vi "Measurement Logic.vi"() -> ()   [LabVIEW 2023, in "NIDCPowerSourceDCVoltage.lvlib"]
uses:
  NIDCPowerSourceDCVoltage.lvlib
  Measurement Configuration.ctl
  Measurement Results.ctl
  <vilib>/Plug-In SDKs/Measurements/Measure Call Context/Measure Call Context.lvclass
  <vilib>/gRPC/Generated APIs/ni/measurementlink/discovery/v1/RPC Messages/ni_measurementlink_discovery_v1_ResolveServiceRequest.ctl
  <vilib>/Plug-In SDKs/Clients/Session Management V1/Session Reservation/Session Reservation.lvclass
  <vilib>/Plug-In SDKs/Sessions/niDCPower/NI Session Management niDCPower.lvlib
  NIDCPowerSourceDCVoltage_client/NIDCPowerSourceDCVoltage_client.lvlib
  <vilib>/Plug-In SDKs/Clients/Discovery V1/NI Discovery V1 Client.lvlib
  <vilib>/gRPC/Generated APIs/ni/measurementlink/discovery/v1/ni.measurementlink.discovery.v1.api.lvlib
panel:
  in  "error in":errorcluster
  in  "request data":T1
  out "error out":errorcluster
  out "measure call context out":refnum<class "Measure Call Context.lvclass">
  in  "measure call context in":refnum<class "Measure Call Context.lvclass">
  out "measurement results":T2
  in  "measurement configuration":T3={"pin_names"=[], "voltage_level"=6.0, "voltage_level_range"=6.0, "current_limit"=0.01, "current_limit_range"=0.01, "source_delay"=0.0}
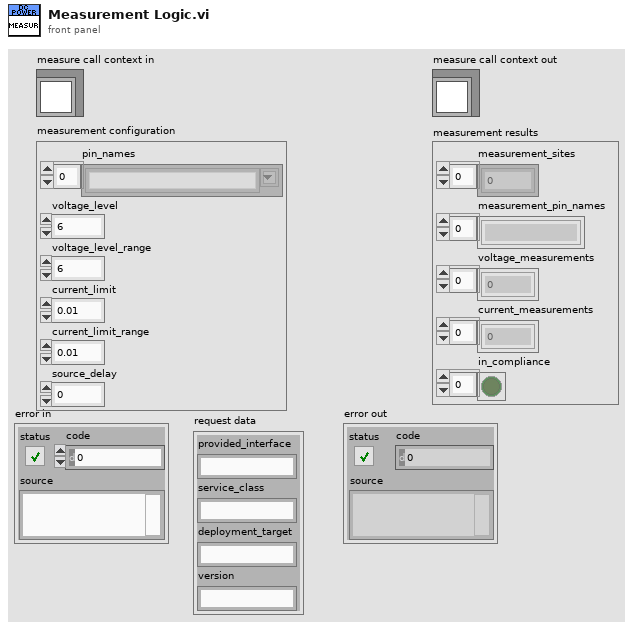
[diagram p1: front panel]
types:
  T1 = typedef "ni.measurementlink.discovery.v1.api.lvlib/ni_measurementlink_discovery_v1_ResolveServiceRequest.ctl" = cluster{"provided_interface":string, "service_class":string, "deployment_target":string, "version":string}
  T2 = typedef "NIDCPowerSourceDCVoltage.lvlib/Measurement Results.ctl" = cluster{"measurement_sites":i32[], "measurement_pin_names":string[], "voltage_measurements":dbl[], "current_measurements":dbl[], "in_compliance":bool[]}
  T3 = typedef "NIDCPowerSourceDCVoltage.lvlib/Measurement Configuration.ctl" = cluster{"pin_names":string[], "voltage_level":dbl, "voltage_level_range":dbl, "current_limit":dbl, "current_limit_range":dbl, "source_delay":dbl}
  T4 = typedef "ni.measurementlink.discovery.v1.api.lvlib/ni_measurementlink_discovery_v1_ServiceLocation.ctl" = cluster{"location":string, "insecure_port":string, "ssl_authenticated_port":string}
  T5 = typedef "grpc-lvsupport-release.lvlib/grpcId.ctl" = u64
  T6 = typedef "NI Session Management niDCPower.lvlib/Connection with Session.ctl" = cluster{"connection":T7, "session":refnum<k15>}
  T7 = typedef "NI Session Management V1 Client.lvlib/Session Reservation.lvclass/Connection.ctl" = cluster{"pin or relay name":string, "site":i32, "instrument type id":string, "channel":string}
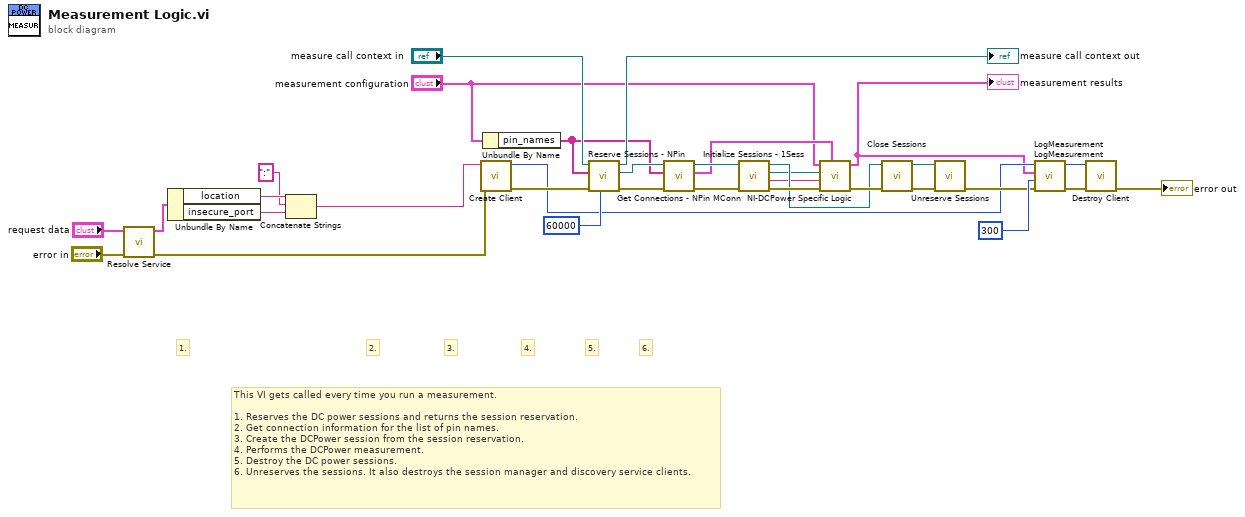
[diagram p0: block diagram]
diagram:
  # "6."
  # "This VI gets called every time you run a measurement.\n\n1. Reserves the DC power sessions and returns the session reservation.\n2. Get connection information for the list of pin names.\n3. Create the DCPower session from the session reservation.\n4. Performs the DCPower measurement.\n5. Destroy the DC power sessions.\n6. Unreserves the sessions. It also destroys the session manager and discovery service clients."
  # "5."
  # "4."
  # "3."
  # "2."
  # "1."
  n1 = call <vilib>:"Resolve Service.vi"("error in"="error in", "request data"="request data") -> ("error out"=w1:errorcluster, "response data"=w6:T4)  [unwired: 8 in]
  n2 = Unbundle By Name(w6) -> ("location"=w5:string, "insecure_port"=w3:string)
  n3 = Concatenate Strings(w5, ":" ("string"), w3) -> (w2:string)
  n4 = call "Create Client.vi"("error in"=w1, "address"=w2) -> ("error out"=w16:errorcluster, "gRPC ID Out"=w11:T5)  [unwired: 8 in]
  n5 = Unbundle By Name("measurement configuration") -> ("pin_names"=w22:string[])
  n6 = call <vilib>:"Reserve Sessions - NPin.vi"("timeout (ms)"=60000, "error in"=w16, "pin or relay names"=w22, "measurement context in"="measure call context in") -> ("error out"=w25:errorcluster, "session reservation out"=w23:refnum<class "Session Reservation.lvclass">, "measurement context out"=→"measure call context out":refnum<class "Measure Call Context.lvclass">)  [unwired: 5 in]
  n7 = call <vilib>:"Get Connections - NPin MConn.vi"("error in"=w25, "pin or relay names"=w22, "session reservation in"=w23) -> ("error out"=w24:errorcluster, "connections"=w20:T6[], "session reservation out"=w21:refnum<class "Session Reservation.lvclass">)  [unwired: 6 in]
  n8 = call <vilib>:"Initialize Sessions - 1Sess.vi"("error in"=w24, "session reservation in"=w21) -> ("error out"=w33:errorcluster, "channel list"=w18:string, "session"=w19:refnum<k15>, "session reservation out"=w29:refnum<class "Session Reservation.lvclass">)  [unwired: 6 in]
  n9 = call "NI-DCPower Specific Logic.vi"("connections"=w20, "error in"=w33, "channel list"=w18, "instrument handle"=w19, "Measurement Configuration"="measurement configuration") -> ("error out"=w32:errorcluster, "Measurement Results"=w9:T2)  [unwired: 4 in, 1 out]
  "measurement results" <- w9
  n10 = call <vilib>:"Close Sessions.vi"("error in"=w32, "session reservation in"=w29) -> ("error out"=w31:errorcluster, "session reservation out"=w30:refnum<class "Session Reservation.lvclass">)  [unwired: 8 in]
  n11 = call <vilib>:"Unreserve Sessions.vi"("error in"=w31, "session reservation in"=w30) -> ("error out"=w12:errorcluster)  [unwired: 9 in]
  n12 = call "LogMeasurement LogMeasurement.vi"("error in"=w12, "timeout (ms)"=300, "Request Data"=w9, "gRPC ID"=w11) -> ("error out"=w13:errorcluster, "gRPC ID out"=w14:T5)  [unwired: 5 in, 1 out]
  n13 = call "Destroy Client.vi"("error in"=w13, "gRPC ID"=w14) -> ("error out"=→"error out":errorcluster)  [unwired: 9 in]
